vi "LvMPDC_SUB_convert_pathtext2path.vi"(10 "pathtext":string) -> (2 "path":path)   [LabVIEW 2012]
panel:
  # "file:"
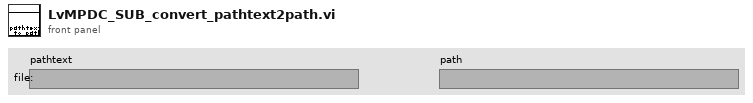
[diagram p1: front panel]
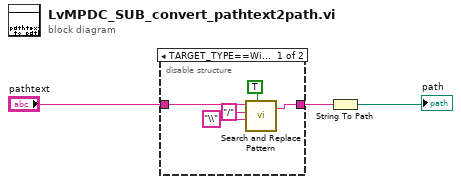
[diagram p0: block diagram]
diagram:
  n1 = disable-structure shown="TARGET_TYPE==Windows" {
    disable-tunnel: "pathtext" -> [w7 w9]
    disable-tunnel: [w4 w9] -> w2
    frame condition #0 (active) {
      n2 = call <vilib>:"Search and Replace Pattern.vi"("string"=w7, "regular expression (\"\")"="/" ("regular expression (\"\")"), "replace string (\"\")"="\\" ("replace string (\"\")"), "replace all? (F)"=TRUE) -> ("result string"=w4:string)  [unwired: 1 in, 1 out]
    }
    frame condition #1 {
    }
  }
  n3 = String To Path(string=w2) -> (path=→"path":path)
